vi "Control Arm Sholder APP V2.vi"() -> ()   [LabVIEW 2015]
uses:
  Global Distance.vi
  Global Angle.vi
panel:
  in  "z limit":dbl=1.0 format="%#_13g"
  in  "Grip":bool
  in  "statee":dbl
  in  "stop 3":bool
  in  "dy input 2":dbl
  in  "dz input":dbl(slide) scale=0.0..130.0
  out "delta3":dbl
  in  "stop 2":bool
  out "x*y":dbl
  in  "Boolean 2":bool
  out "delta2":dbl
  out "delta1":dbl
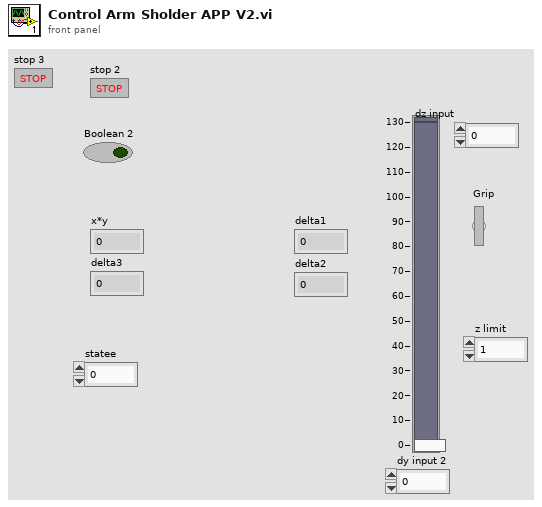
[diagram p1: front panel]
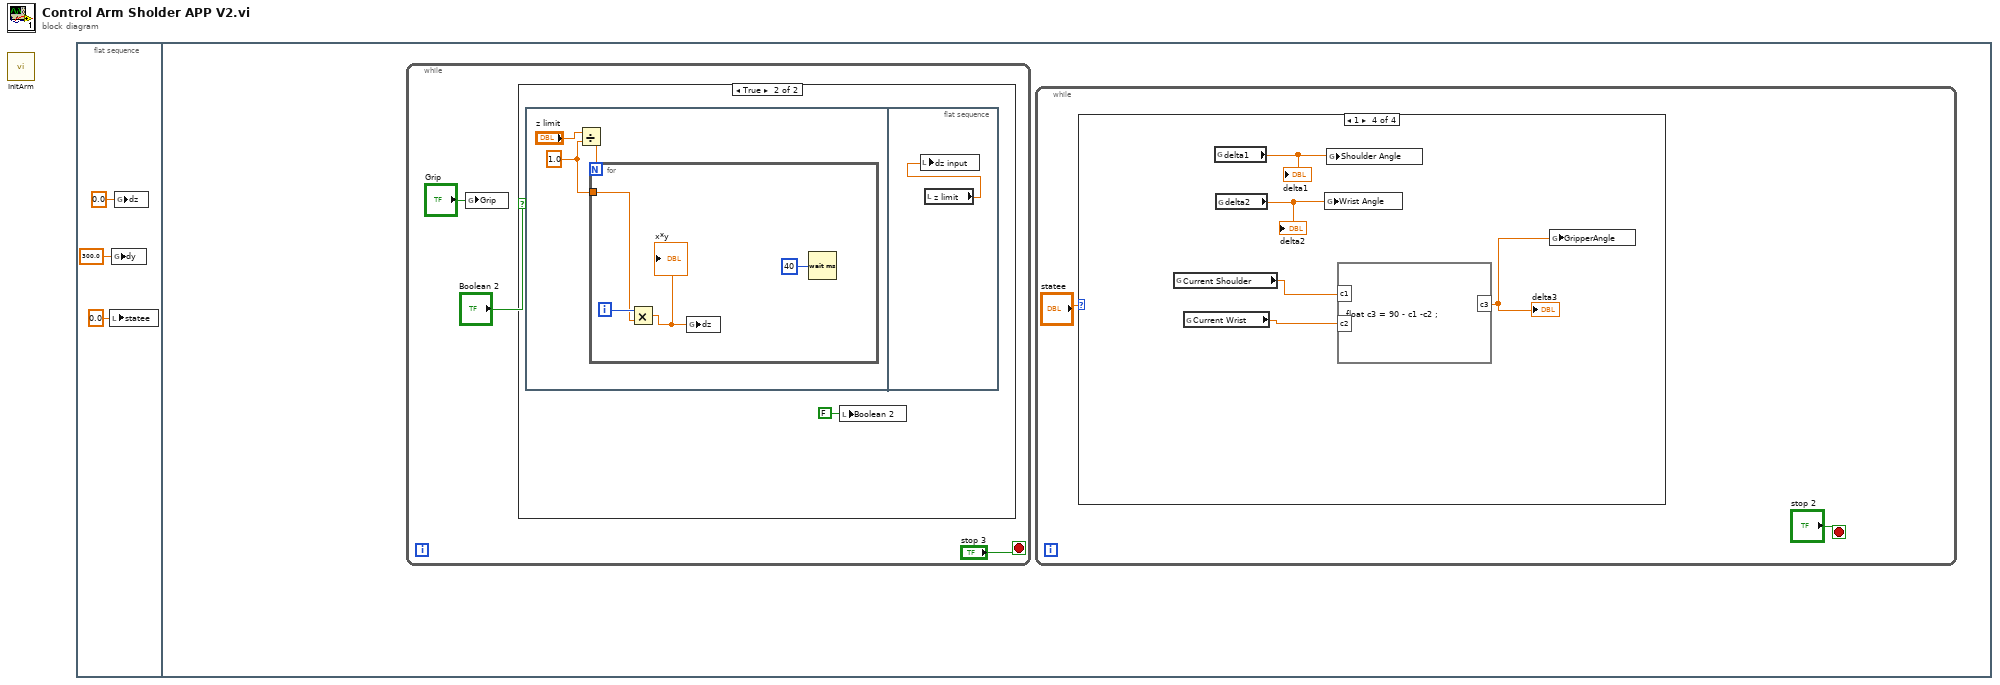
[diagram p0: block diagram]
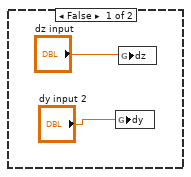
[diagram p2: hidden frame]
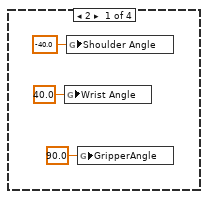
[diagram p3: hidden frame]
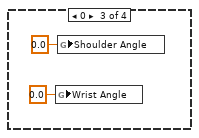
[diagram p5: hidden frame]
diagram:
  n1 = call "InitArm.vi"() -> ()  [unwired: 12 in]
  n2 = flat-sequence {
    frame #0 {
      n3 = local write "statee"(0.0 ("statee")) -> ()
      n4 = global write "Global Distance.vi" "dy"(300.0 ("dy")) -> ()
      n5 = global write "Global Distance.vi" "dz"(0.0 ("dz")) -> ()
    }
    frame #1 {
      n6 = while {
        stop <- "stop 3" stop-if-true
        n7 = global write "Global Angle.vi" "Grip"("Grip") -> ()
        n8 = case shown="True" "Boolean 2" {
          frame False {
            n9 = global write "Global Distance.vi" "dy"("dy input 2") -> ()
            n10 = global write "Global Distance.vi" "dz"("dz input") -> ()
          }
          frame True {
            n11 = flat-sequence {
              frame #0 {
                w10 = 1.0 ("y")
                n12 = Divide(x="z limit", y=w10) -> (x/y=w12:dbl)
                n13 = for {
                  N: w12 -> [_]
                  tunnel: w10 -> [w13]
                  i -> [w15]
                  n14 = Multiply(x=w15, y=w13) -> (x*y=w14:dbl)
                  "x*y" <- w14
                  n15 = global write "Global Distance.vi" "dz"(w14) -> ()
                  n16 = Wait (ms)(milliseconds to wait=u32 40) -> ()  [unwired: 1 out]
                }
              }
              frame #1 {
                n17 = local read "z limit"() -> (w17:dbl)
                n18 = local write "dz input"(w17) -> ()
              }
            }
            n19 = local write "Boolean 2"(FALSE ("Boolean 2")) -> ()
          }
        }
      }
      n20 = while {
        stop <- "stop 2" stop-if-true
        n21 = case shown="1" "statee" {
          frame 2 {
            n22 = global write "Global Angle.vi" "Wrist Angle"(40.0 ("Wrist Angle")) -> ()
            n23 = global write "Global Angle.vi" "Shoulder Angle"(-40.0 ("Shoulder Angle")) -> ()
            n24 = global write "Global Angle.vi" "GripperAngle"(90.0 ("GripperAngle")) -> ()
          }
          frame 3, Default {
          }
          frame 0 {
            n25 = global write "Global Angle.vi" "Wrist Angle"(0.0 ("Wrist Angle")) -> ()
            n26 = global write "Global Angle.vi" "Shoulder Angle"(0.0 ("Shoulder Angle")) -> ()
          }
          frame 1 {
            n27 = global read "Global Angle.vi" "Current Shoulder"() -> (w27:dbl)
            n28 = global read "Global Angle.vi" "Current Wrist"() -> (w26:dbl)
            n29 = global read "Global Distance.vi" "delta1"() -> (w29:dbl)
            "delta1" <- w29
            n30 = global read "Global Distance.vi" "delta2"() -> (w28:dbl)
            "delta2" <- w28
            n31 = global write "Global Angle.vi" "Wrist Angle"(w28) -> ()
            n32 = global write "Global Angle.vi" "Shoulder Angle"(w29) -> ()
            n33 = formula code="float c3 = 90 - c1 -c2 ;"("c1"=w27, "c2"=w26) -> ("c3"=w25:dbl)
            "delta3" <- w25
            n34 = global write "Global Angle.vi" "GripperAngle"(w25) -> ()
          }
        }
      }
    }
  }
